vi "T Deg F to Deg C.vi"() -> ()   [LabVIEW 2024]
panel:
  out "T (C)":dbl
  in  "T (F)":dbl
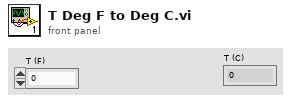
[diagram p1: front panel]
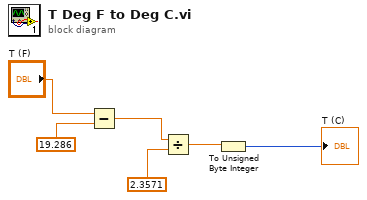
[diagram p0: block diagram]
diagram:
  n1 = Subtract(x="T (F)", y=19.286) -> (x-y=w4:dbl)
  n2 = Divide(x=w4, y=2.3571) -> (x/y=w2:dbl)
  n3 = To Unsigned Byte Integer(number=w2) -> (unsigned 8bit integer=→"T (C)":u8)
